vi "ProcessHandshakeRequest.vi"(8 "error in (no error)":errorcluster, 11 "HTTP Headers":string) -> (0 "error out":errorcluster, 1 "Sec-WebSocket-Key":string, 2 "Path":string, 3 "Is Websocket Request?":bool, 4 "Headers Out":variant, 5 "Host":string)   [LabVIEW 2014, in "QwaveSys RPi Training Library.lvlib" / "WebSockets.lvlib"]
doc: "WebSockets API 1.3.0.13\nSam Sharp - Intelligent Energy\nCopyright (c) 2015, Intelligent Energy"
uses:
  <vilib>/Q-Wave Systems/QwaveSys RPi Package 2.0/Addons/WebSockets API/WebSockets/WebSockets.lvlib
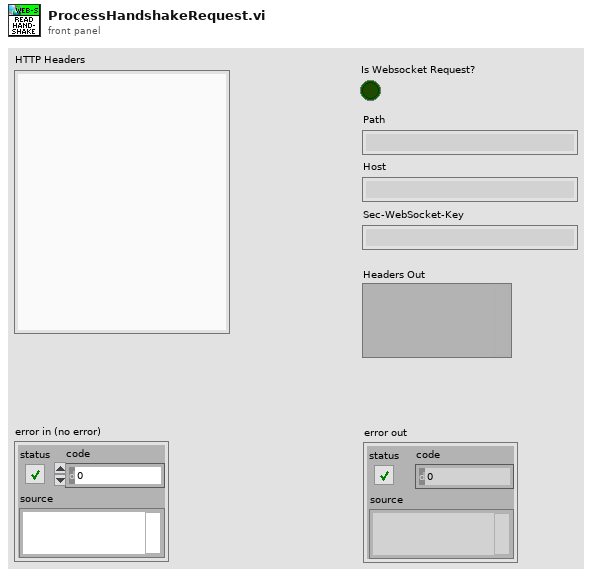
[diagram p1: front panel]
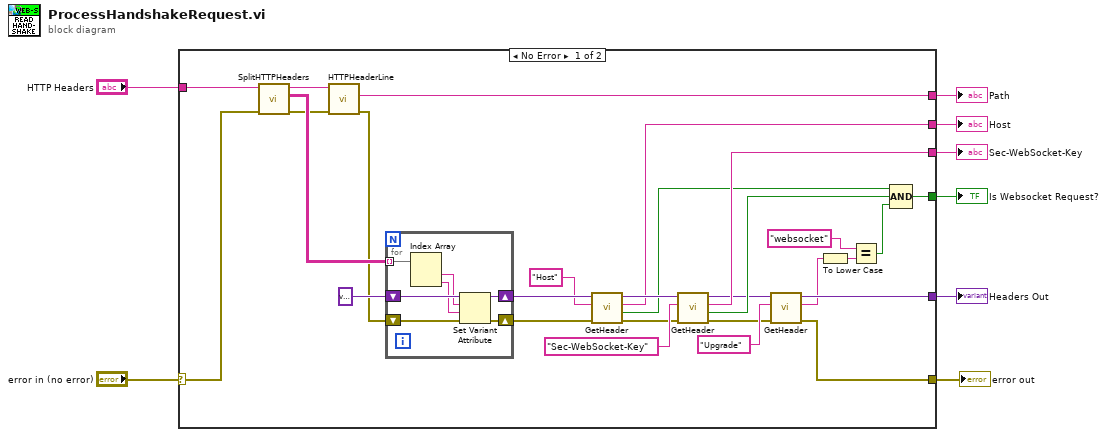
[diagram p0: block diagram]
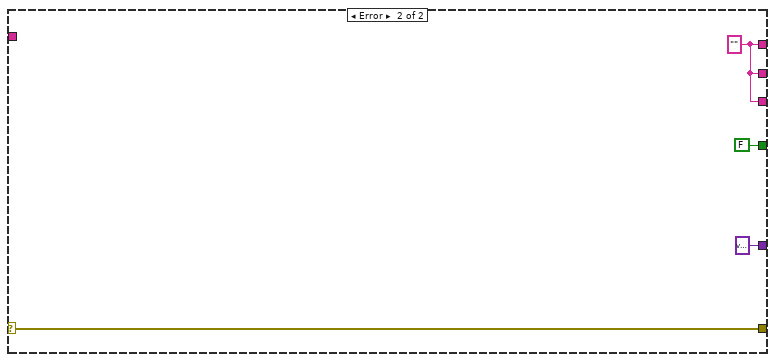
[diagram p2: hidden frame]
diagram:
  n1 = case shown="No Error" "error in (no error)" {
    selector: "error in (no error)" -> [w17 w47]
    tunnel: "HTTP Headers" -> [w36 _]
    tunnel: [w32 w45] -> w7
    tunnel: [w28 w45] -> w6
    tunnel: [w26 w45] -> w5
    tunnel: [w22 variant ("Headers Out")] -> w4
    tunnel: [w18 FALSE] -> w3
    tunnel: [w13 w47] -> w1
    frame No Error {
      n2 = call <vilib>:"SplitHTTPHeaders.vi"("error in (no error)"=w17, "HTTP Header String"=w36) -> ("error out"=w16:errorcluster, "Headers Array"=w34:string[][], "HTTP Request"=w35:string)  [unwired: 7 in]
      n3 = call <vilib>:"HTTPHeaderLine.vi"("error in (no error)"=w16, "HTTP Request Line"=w35) -> ("error out"=w11:errorcluster, "Request URI"=w32:string)  [unwired: 6 in, 2 out]
      n4 = for {
        tunnel: w34 -> [w43] mode=indexing
        shift-right: [w41] -> w31
        shift-left: variant -> [w42]
        shift-right: [w38] -> w12
        shift-left: w11 -> [w37]
        n5 = Index Array(array=w43) -> (element #1=w40:string, element #2=w39:string)  [unwired: 2 in]
        n6 = Set Variant Attribute(Variant=w42, name=w40, value=w39, error in=w37) -> (Variant out=w41:variant, error out=w38:errorcluster)  [unwired: 1 out]
      }
      n7 = call <vilib>:"GetHeader.vi"("error in (no error)"=w12, "Name"="Host" ("name"), "Headers In"=w31) -> ("error out"=w15:errorcluster, "Found?"=w25:bool, "Data"=w28:string, "Headers Out"=w29:variant)  [unwired: 5 in]
      n8 = call <vilib>:"GetHeader.vi"("error in (no error)"=w15, "Name"="Sec-WebSocket-Key", "Headers In"=w29) -> ("error out"=w14:errorcluster, "Found?"=w24:bool, "Data"=w26:string, "Headers Out"=w23:variant)  [unwired: 5 in]
      n9 = call <vilib>:"GetHeader.vi"("error in (no error)"=w14, "Name"="Upgrade", "Headers In"=w23) -> ("error out"=w13:errorcluster, "Data"=w10:string, "Headers Out"=w22:variant)  [unwired: 5 in, 1 out]
      n10 = To Lower Case(string=w10) -> (all lower case string=w9:string)
      n11 = Equal?(x="websocket", y=w9) -> (x = y?=w19:bool)
      n12 = Compound Arithmetic op=AND(w25, w24, w19) -> (w18:bool)
    }
    frame Error {
      w45 = "" ("Request URI")
    }
  }
  "Host" <- w6
  "Path" <- w7
  "Sec-WebSocket-Key" <- w5
  "Is Websocket Request?" <- w3
  "Headers Out" <- w4
  "error out" <- w1
